vi "ke37xx DMM Configuration.vi"(0 "VISA Resource Name":refnum<visa-resource-name>, 5 "Configuration Name":string, 11 "error in (no error)":errorcluster, 12 "Bytes To Read (1024)":u32=1024) -> (4 "VISA Resource Name Out":refnum<visa-resource-name>, 8 "Configuration Settings":string[](array[string]), 15 "error out":errorcluster)   [LabVIEW 2009, in "Keithley 3700 Series.lvlib"]
doc: "This VI allows you to create, delete, recall, and query DMM configurations. A DMM configuration consists of the currently selected measurement function as well as all pertinent DMM attributes. These settings are associated with a named configuration that can be recalled to configure the DMM in specific ways."
uses:
  <instrlib>/Keithley 3706/Keithley 3700 Series.lvlib
panel:
  in  "Action":enum16{"Create", "Delete", "Recall", "Query"}(ring)
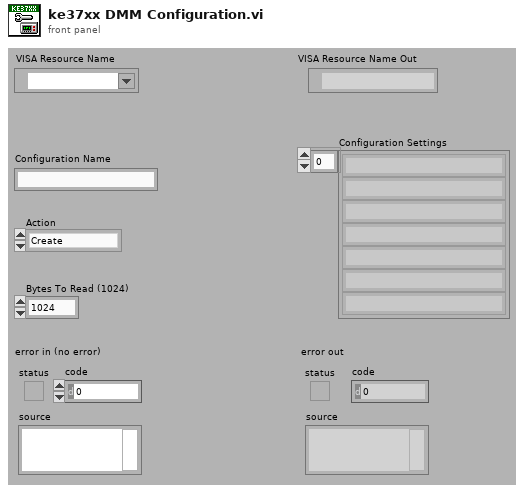
[diagram p1: front panel]
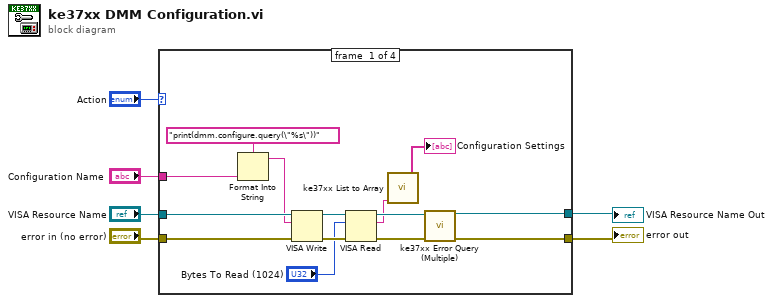
[diagram p0: block diagram]
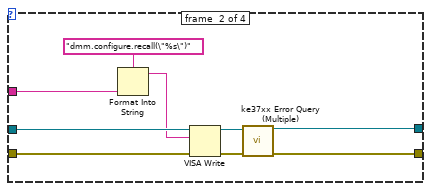
[diagram p2: hidden frame]
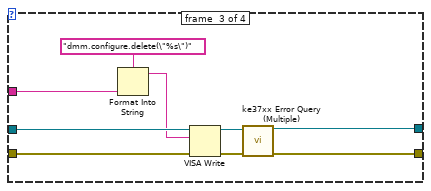
[diagram p3: hidden frame]
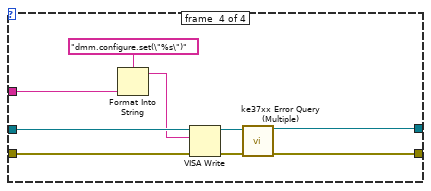
[diagram p4: hidden frame]
diagram:
  n1 = case shown="\"Query\"" "Action" {
    tunnel: [w20 w29 w38 w47] -> w6
    tunnel: [w19 w28 w37 w46] -> w5
    tunnel: "VISA Resource Name" -> [w17 w26 w35 w44]
    tunnel: "error in (no error)" -> [w16 w25 w34 w43]
    tunnel: "Configuration Name" -> [w11 w24 w33 w42]
    frame #0 {
      n2 = Format Into String(format string="print(dmm.configure.query(\"%s\"))", w11) -> (resulting string=w10:string)  [unwired: 2 in, 1 out]
      n3 = VISA Write(VISA resource name=w17, write buffer=w10, error in (no error)=w16) -> (VISA resource name out=w15:refnum<visa-resource-name>, error out=w13:errorcluster)  [unwired: 1 out]
      n4 = VISA Read(VISA resource name=w15, byte count="Bytes To Read (1024)", error in (no error)=w13) -> (VISA resource name out=w14:refnum<visa-resource-name>, read buffer=w8:string, error out=w12:errorcluster)  [unwired: 1 out]
      n5 = call <instrlib>:"ke37xx List to Array.vi"("List"=w8) -> ("Output String Array"=→"Configuration Settings":string[])  [unwired: 1 in, 5 out]
      n6 = call <instrlib>:"ke37xx Error Query (Multiple).vi"("VISA resource name"=w14, "error in (no error)"=w12) -> ("VISA resource name out"=w20:refnum<visa-resource-name>, "error out"=w19:errorcluster)  [unwired: 12 out]
    }
    frame #1 {
      n7 = Format Into String(format string="dmm.configure.recall(\"%s\")", w24) -> (resulting string=w23:string)  [unwired: 2 in, 1 out]
      n8 = VISA Write(VISA resource name=w26, write buffer=w23, error in (no error)=w25) -> (VISA resource name out=w22:refnum<visa-resource-name>, error out=w21:errorcluster)  [unwired: 1 out]
      n9 = call <instrlib>:"ke37xx Error Query (Multiple).vi"("VISA resource name"=w22, "error in (no error)"=w21) -> ("VISA resource name out"=w29:refnum<visa-resource-name>, "error out"=w28:errorcluster)  [unwired: 12 out]
    }
    frame #2 {
      n10 = Format Into String(format string="dmm.configure.delete(\"%s\")", w33) -> (resulting string=w32:string)  [unwired: 2 in, 1 out]
      n11 = VISA Write(VISA resource name=w35, write buffer=w32, error in (no error)=w34) -> (VISA resource name out=w31:refnum<visa-resource-name>, error out=w30:errorcluster)  [unwired: 1 out]
      n12 = call <instrlib>:"ke37xx Error Query (Multiple).vi"("VISA resource name"=w31, "error in (no error)"=w30) -> ("VISA resource name out"=w38:refnum<visa-resource-name>, "error out"=w37:errorcluster)  [unwired: 12 out]
    }
    frame #3 {
      n13 = Format Into String(format string="dmm.configure.set(\"%s\")", w42) -> (resulting string=w41:string)  [unwired: 2 in, 1 out]
      n14 = VISA Write(VISA resource name=w44, write buffer=w41, error in (no error)=w43) -> (VISA resource name out=w40:refnum<visa-resource-name>, error out=w39:errorcluster)  [unwired: 1 out]
      n15 = call <instrlib>:"ke37xx Error Query (Multiple).vi"("VISA resource name"=w40, "error in (no error)"=w39) -> ("VISA resource name out"=w47:refnum<visa-resource-name>, "error out"=w46:errorcluster)  [unwired: 12 out]
    }
  }
  "VISA Resource Name Out" <- w6
  "error out" <- w5
